vi "KE2657A_CommandsGlobal.vi"() -> ()   [LabVIEW 2018, in "KE2657A.lvclass"]
uses:
  KE2657A.lvclass
panel:
  in  "Keithley 2657A GPIB Setup":T1={"Instrument name"="Keithley 2657A", "Command \"Reset\""="smua.reset()", "Command \"Initialise\""="smua.trigger.count = 0\nsmua.source.func = OUTPUT_DCVOLTS\nsmua.source.rangev = 700\nsmua.source.limiti = 10E-06\nsmua.source.autorangev = smua.AUTORANGE_ON\nsmua.measure.autorangei = smua.AUTORANGE_ON", "Command \"Arm\""="smua.source.output = smua.OUTPUT_OFF\nsmua.measure.autozero = smua.AUTOZERO_ONCE \nsmua.source.levelv = 0 \nsmua.source.output = smua.OUTPUT_ON", "Command \"SetVolts\""="smua.source.levelv = %3.2f", "Command \"Compliance?\""="compliance = smua.source.compliance\nprint(compliance)", "Command \"Standby\""="smua.source.levelv = 0\nsmua.measure.autozero = smua.AUTOZERO_AUTO\nsmua.source.output = smua.OUTPUT_OFF", "Command \"Read Current\""="print(smua.measure.i())"}
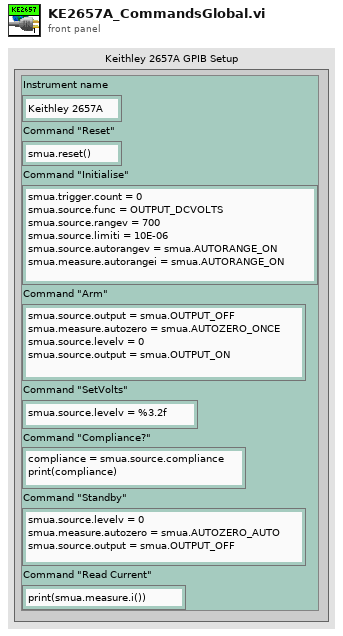
[diagram p1: front panel]
types:
  T1 = cluster{"Instrument name":string, "Command \"Reset\"":string, "Command \"Initialise\"":string, "Command \"Arm\"":string, "Command \"SetVolts\"":string, "Command \"Compliance?\"":string, "Command \"Standby\"":string, "Command \"Read Current\"":string}
diagram:
